vi "AI 9234-Acclerometer Test.vi"() -> ()   [LabVIEW 2021]
uses:
  <vilib>/DAQmx/read.llb/DAQmx Read (Analog 1D Wfm NChan NSamp).vi
  <vilib>/DAQmx/create/channels.llb/DAQmx Create Channel (AI-Acceleration-Accelerometer).vi
  <vilib>/DAQmx/configure/timing.llb/DAQmx Timing (Sample Clock).vi
  <vilib>/DAQmx/miscellaneous.llb/DAQmx Fill In Error Info.vi
  <resource>/objmgr/daqmx.rc
panel:
  in  "minimum value":dbl=-5.0 format="%0.2f"
  in  "maximum value":dbl=5.0 format="%0.2f"
  in  "current excitation value":dbl=0.004
  in  "current excitation source":i32(ring)=10200 items=["Internal"=10200, "External"=10167, "None"=10230]
  in  "sensitivity units":i32(ring)=12509 items=["mVolts/g"=12509, "Volts/g"=12510]
  in  "sensitivity":dbl=1000.0
  in  "units":i32(ring)=10186 items=["g"=10186, "m/s^2"=12470, "in/s^2"=12471, "From Custom Scale"=10065]
  in  "input terminal configuration":i32(ring)=-1 items=["default"=-1, "RSE"=10083, "NRSE"=10078, "Differential"=10106, "Pseudodifferential"=12529]
  in  "error in (no error)":errorcluster
  out "SampClk.Rate":dbl
  out "Configuring Channel":tag[](array[tag])
  out "Actual Sampling Rate":dbl
  out "Timing.samples per channel":i32
  out "ms  to Wait":u32
  in  "rate":dbl=1000.0 format="%0.2f"
  in  "samples per channel":i32=1000
  in  "sample mode":i32(ring)=10178 items=["Finite Samples"=10178, "Continuous Samples"=10123, "Hardware Timed Single Point"=12522]
  out "AI.PhysicalChans":tag[](array[tag])
  in  "Stop":bool
  out "data":waveform(dbl)[](array[waveform])
  out "Waveform Chart":waveform(dbl)[](graph)
  out "Waveform Graph":waveform(dbl)[](graph)
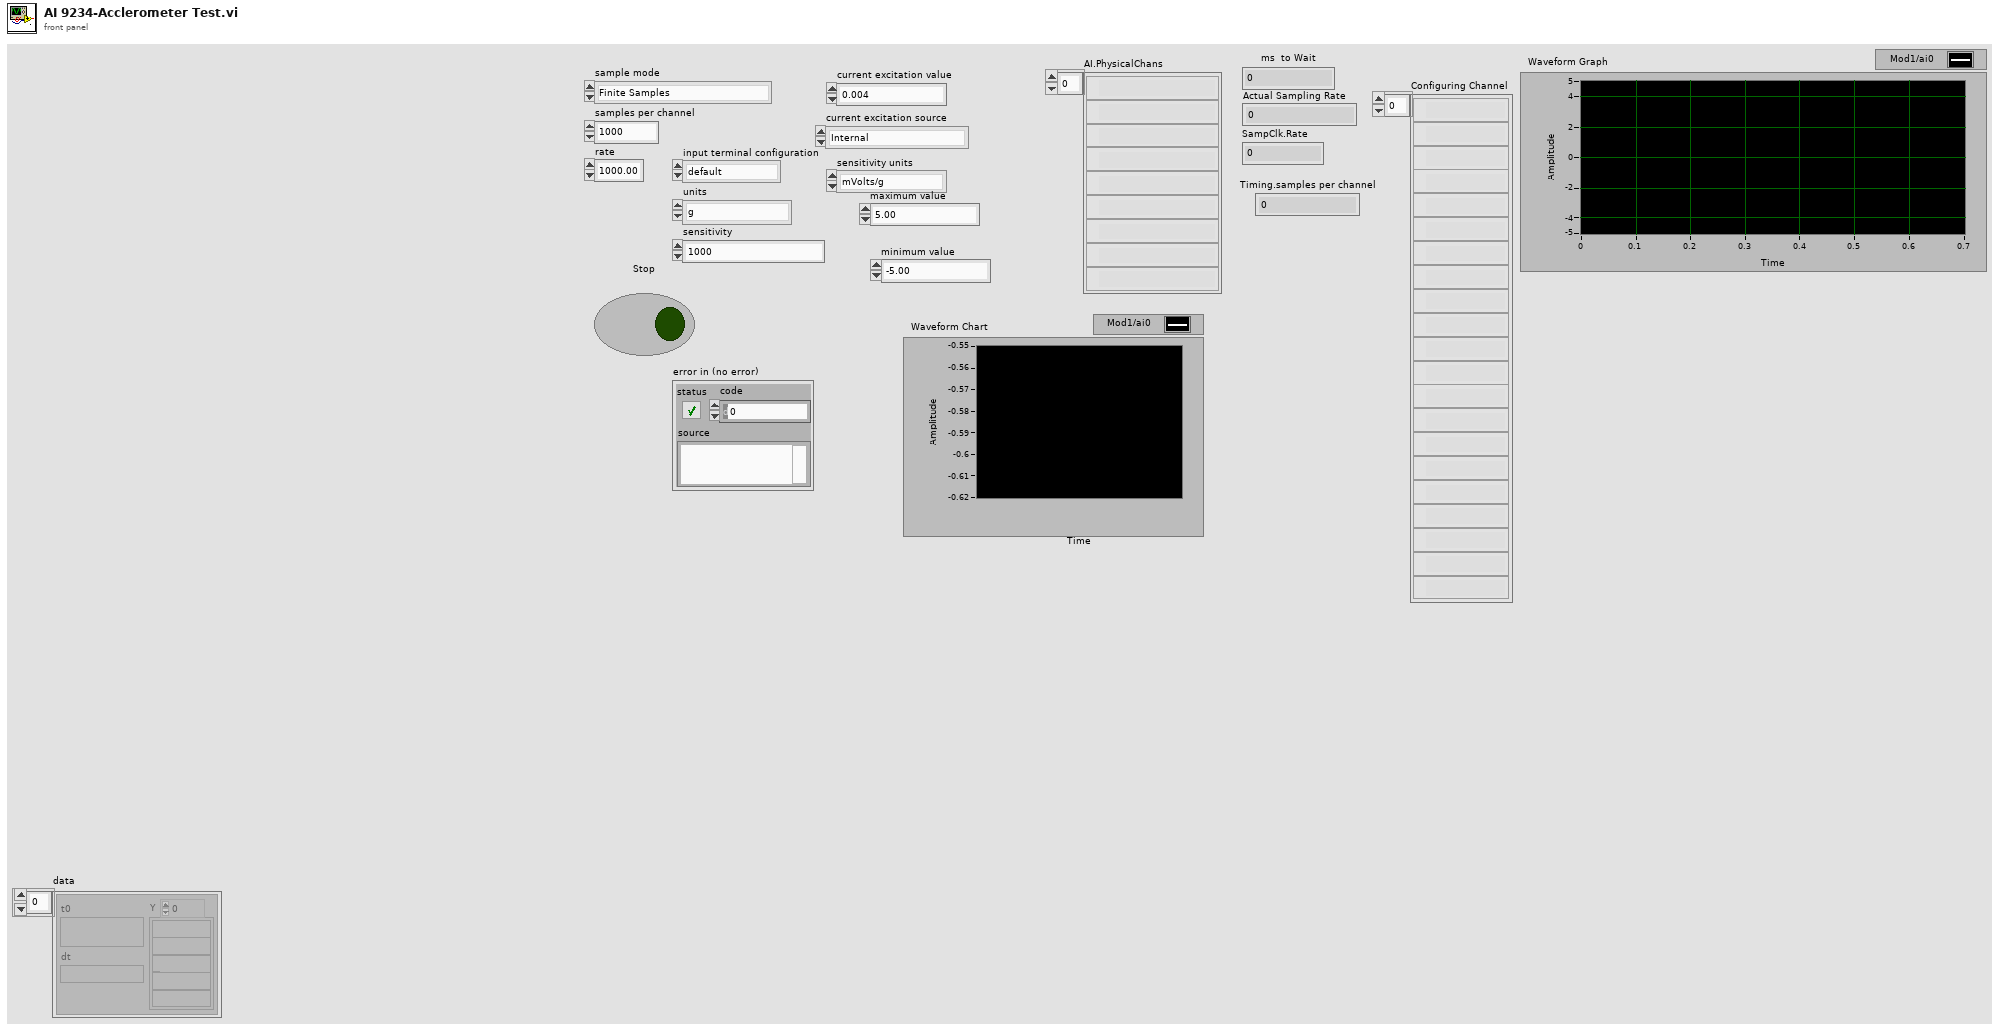
[diagram p1: front panel]
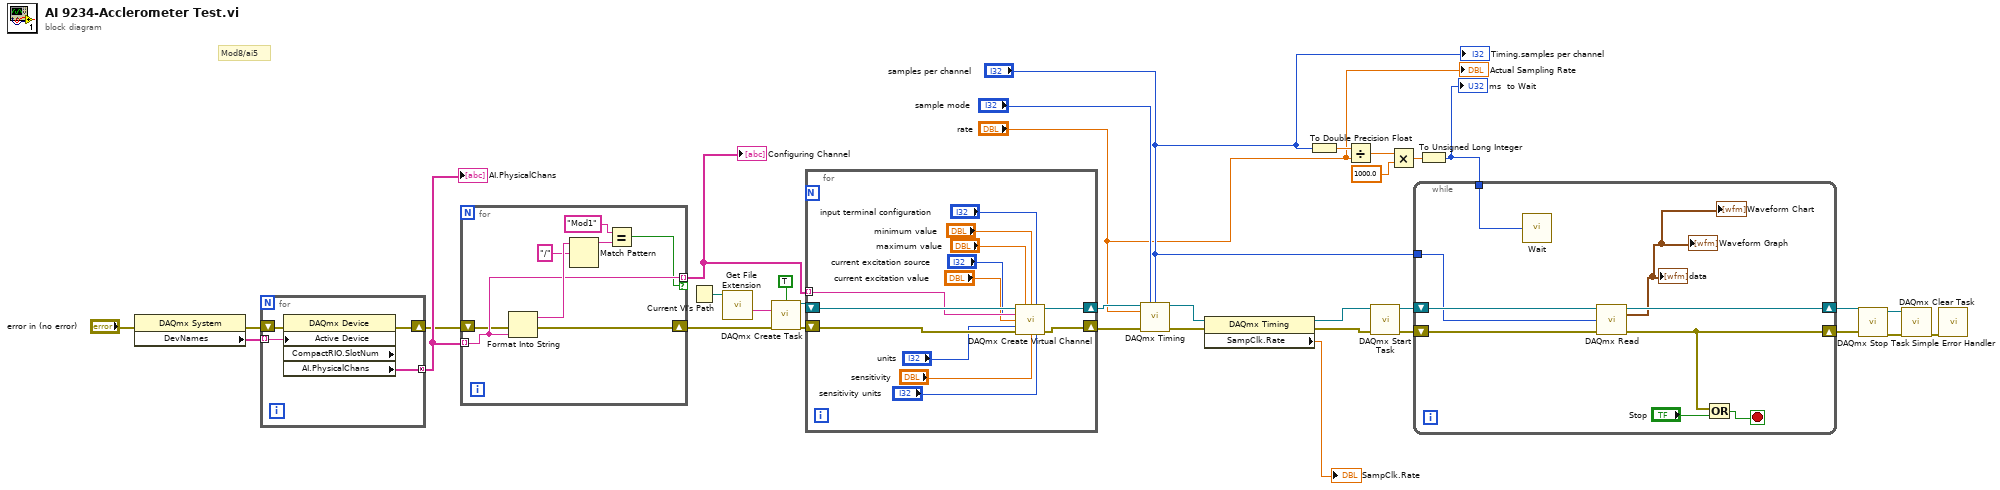
[diagram p0: block diagram]
diagram:
  # "Mod8/ai5"
  n1 = property class="DAQmx System"(error in="error in (no error)") -> (error out=w30:errorcluster, "DevNames"=w34:tag[])  [unwired: 1 in, 1 out]
  n2 = for {
    tunnel: w34 -> [w38] mode=indexing
    shift-right: [w37] -> w4
    shift-left: w30 -> [w36]
    tunnel: [w35] -> w12 mode=concatenating
    n3 = property class="DAQmx Device" props=["Active Device", "CompactRIO.SlotNum", "AI.PhysicalChans"](error in=w36, "Active Device"=w38) -> (error out=w37:errorcluster, "AI.PhysicalChans"=w35:tag[])  [unwired: 1 in, 2 out]
  }
  "AI.PhysicalChans" <- w12
  n4 = for {
    tunnel: w12 -> [w42] mode=indexing
    tunnel: [w42] -> w11 mode=indexing if=w41
    shift-right: [w39] -> w3
    shift-left: w4 -> [w40]
    n5 = Format Into String(error in=w40, w42) -> (resulting string=w46:string, error out=w39:errorcluster)  [unwired: 2 in]
    n6 = Match Pattern(string=w46, regular expression="/") -> (before substring=w44:string)  [unwired: 1 in, 3 out]
    n7 = Equal?(x="Mod1" ("regular expression"), y=w44) -> (x = y?=w41:bool)
  }
  "Configuring Channel" <- w11
  n8 = Current VI's Path() -> (path=w2:path)
  n9 = call <vilib>:"Get File Extension.vi"("file"=w2) -> ("filename without extension"=w1:string)  [unwired: 6 in, 4 out]
  n10 = call <vilib>:"DAQmx Create Task.vi"("new task name"=w1, "auto cleanup"=TRUE, "error in"=w3) -> ("task out"=w31:refnum<k21>, "error out"=w32:errorcluster)  [unwired: 11 in]
  n11 = for {
    shift-right: [w57] -> w22
    shift-left: w32 -> [w59]
    shift-right: [w56] -> w21
    shift-left: w31 -> [w58]
    tunnel: w11 -> [w55] mode=indexing
    n12 = call-poly <vilib>:"DAQmx Create Virtual Channel.vi"("task in"=w58, "maximum value"="maximum value", "minimum value"="minimum value", "input terminal configuration"="input terminal configuration", "physical channels"=w55, "current excitation source"="current excitation source", "current excitation value"="current excitation value", "units"="units", "error in"=w59, "sensitivity"="sensitivity", "sensitivity units"="sensitivity units") -> ("task out"=w56:refnum<k21>, "error out"=w57:errorcluster)  [unwired: 3 in]
  }
  n13 = call-poly <vilib>:"DAQmx Timing.vi"("task/channels in"=w21, "sample mode"="sample mode", "samples per channel"="samples per channel", "rate"="rate", "error in"=w22) -> ("task out"=w10:refnum<k21>, "error out"=w8:errorcluster)  [unwired: 9 in]
  n14 = property class="DAQmx Timing"(reference=w10, error in=w8) -> (reference out=w6:refnum<k21>, error out=w7:errorcluster, "SampClk.Rate"=→"SampClk.Rate":dbl)
  n15 = To Double Precision Float(number="samples per channel") -> (double precision float=w16:dbl)
  n16 = Divide(x=w16, y="rate") -> (x/y=w18:dbl)
  n17 = call <vilib>:"DAQmx Start Task.vi"("task/channels in"=w6, "error in"=w7) -> ("task out"=w29:refnum<k21>, "error out"=w28:errorcluster)  [unwired: 12 in]
  n18 = Multiply(x=w18, y=1000.0) -> (x*y=w17:dbl)
  n19 = To Unsigned Long Integer(number=w17) -> (unsigned 32bit integer=w13:u32)
  "ms  to Wait" <- w13
  n20 = while {
    shift-right: [w63] -> w24
    shift-left: w29 -> [w66]
    shift-right: [w64] -> w27
    shift-left: w28 -> [w65]
    tunnel: "samples per channel" -> [w62]
    tunnel: w13 -> [w60]
    stop <- w67 stop-if-true
    n21 = call "Wait"("Count(mSec)"=w60) -> ()  [unwired: 1 out]
    n22 = call-poly <vilib>:"DAQmx Read.vi"("task/channels in"=w66, "number of samples per channel"=w62, "error in"=w65) -> ("task out"=w63:refnum<k21>, "data"=→"data" →"Waveform Chart" →"Waveform Graph":waveform(dbl)[], "error out"=w64:errorcluster)  [unwired: 10 in]
    n23 = Or(x=w64, y="Stop") -> (x .or. y?=w67:bool)
  }
  n24 = call <vilib>:"DAQmx Stop Task.vi"("task/channels in"=w24, "error in"=w27) -> ("task out"=w23:refnum<k21>, "error out"=w26:errorcluster)  [unwired: 12 in]
  n25 = call <vilib>:"DAQmx Clear Task.vi"("task in"=w23, "error in"=w26) -> ("error out"=w25:errorcluster)  [unwired: 13 in]
  n26 = call <vilib>:"Simple Error Handler.vi"("error in (no error)"=w25) -> ()  [unwired: 4 in, 5 out]
  "Timing.samples per channel" <- "samples per channel"
  "Actual Sampling Rate" <- "rate"
